vi "Is Connection Error.vi"(8 "error in (no error)":errorcluster, 11 "Instrument.OxfordVRM in":refnum<class "Instrument.OxfordVRM.lvclass">) -> (0 "error out":errorcluster, 2 "Connection Error?":bool, 3 "Instrument.OxfordVRM out":refnum<class "Instrument.OxfordVRM.lvclass">)   [LabVIEW 2019, in "Instrument.OxfordVRM.lvclass"]
uses:
  Instrument.OxfordVRM.lvclass
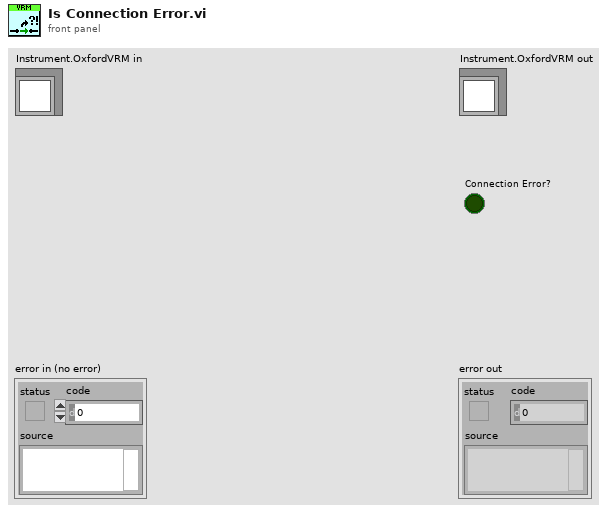
[diagram p1: front panel]
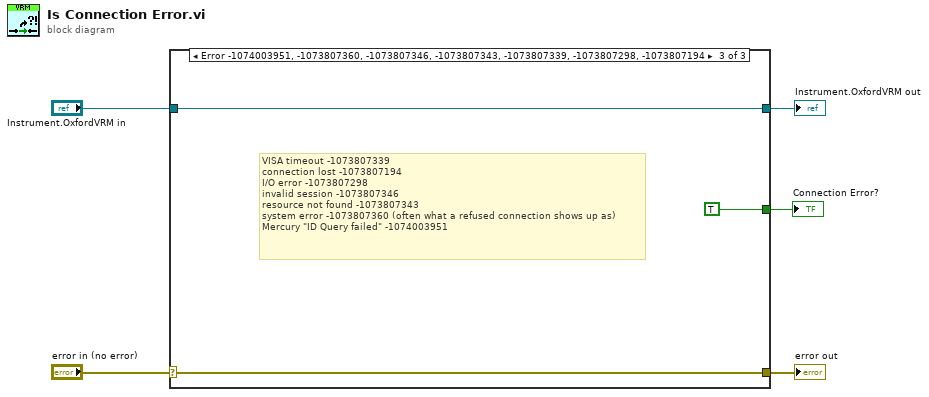
[diagram p0: block diagram]
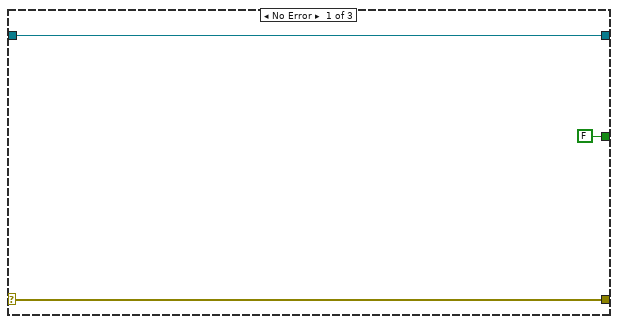
[diagram p2: hidden frame]
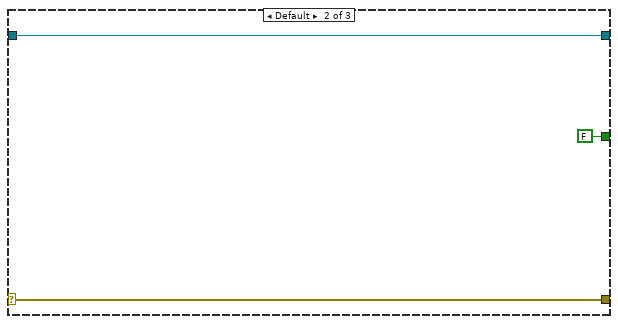
[diagram p3: hidden frame]
diagram:
  n1 = case shown="Error -1074003951, -1073807360, -1073807346, -1073807343, -1073807339, -1073807298, -1073807194" "error in (no error)" {
    selector: "error in (no error)" -> [w7 w11 w14]
    tunnel: [w7 w11 w14] -> w2
    tunnel: [w8 w10 w13] -> w3
    tunnel: "Instrument.OxfordVRM in" -> [w8 w10 w13]
    tunnel: [FALSE ("Connection Error?") FALSE ("Connection Error?") TRUE ("Connection Error?")] -> w5
    frame No Error {
    }
    frame Default {
    }
    frame Error {
      # "VISA timeout -1073807339\nconnection lost -1073807194\nI/O error -1073807298\ninvalid session -1073807346\nresource not found -1073807343\nsystem error -1073807360 (often what a refused connection shows up as)\nMercury \"ID Query failed\" -1074003951"
    }
  }
  "error out" <- w2
  "Instrument.OxfordVRM out" <- w3
  "Connection Error?" <- w5
